vi "JSON Sorter.vi"(10 "Found Token Info":T1(array[cluster]), 11 "names":string[](array[string])) -> (3 "Output":T1(array[cluster]))   [LabVIEW 2019]
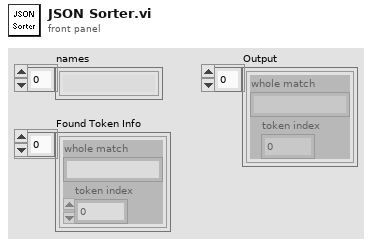
[diagram p1: front panel]
types:
  T1 = cluster{"whole match":string, "token index":i32}[]
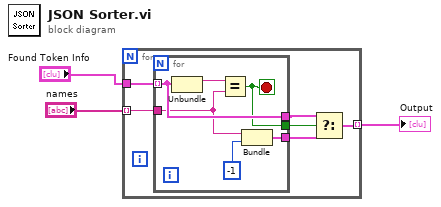
[diagram p0: block diagram]
diagram:
  n1 = for {
    tunnel: "Found Token Info" -> [w9]
    tunnel: "names" -> [w8] mode=indexing
    tunnel: [w5] -> w1 mode=indexing
    n2 = for {
      tunnel: w9 -> [w14] mode=indexing
      tunnel: w8 -> [w11]
      tunnel: [w14] -> w7
      tunnel: [w13] -> w6
      tunnel: [w10] -> w4
      stop <- w13 stop-if-true
      n3 = Unbundle(w14) -> ("whole match"=w15:string)  [unwired: 1 out]
      n4 = Equal?(x=w15, y=w11) -> (x = y?=w13:bool)
      n5 = Bundle("whole match"=w11, "token index"=-1) -> (w10:cluster{"whole match":string, "token index":i32})  [unwired: 1 in]
    }
    n6 = Select(t=w7, s=w6, f=w4) -> (s? t:f=w5:cluster{"whole match":string, "token index":i32})
  }
  "Output" <- w1
